vi "CalcCam4Build.vi"(11 "BuildSize":dbl) -> (3 "CamOut":T1)   [LabVIEW 2014]
uses:
  TypeDefs/Camera.ctl
  <vilib>/Utility/miscctls.llb/LV3DPointTypeDef.ctl
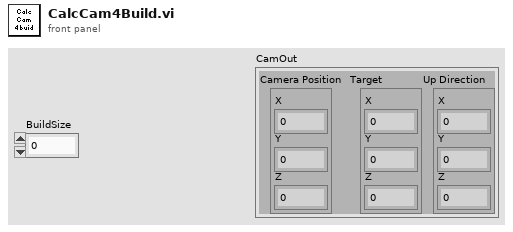
[diagram p1: front panel]
types:
  T1 = typedef "Camera.ctl" = cluster{"Camera Position":T2, "Target":T2, "Up Direction":T2}
  T2 = typedef "LV3DPointTypeDef.ctl" = cluster{"X":sgl, "Y":sgl, "Z":sgl}
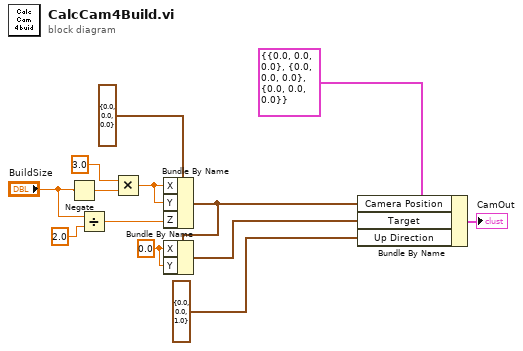
[diagram p0: block diagram]
diagram:
  w10 = sgl 0.0 ("X")
  n1 = Negate(x="BuildSize") -> (-x=w9:dbl)
  n2 = Divide(x="BuildSize", y=2.0) -> (x/y=w11:dbl)
  n3 = Multiply(x=3.0, y=w9) -> (x*y=w7:dbl)
  n4 = Bundle By Name(cluster=T2 {"X"=0.0, "Y"=0.0, "Z"=0.0} ("Camera Position"), "X"=w7, "Y"=w7, "Z"=w11) -> (w5:T2)
  n5 = Bundle By Name(cluster=w5, "X"=w10, "Y"=w10) -> (w4:T2)
  n6 = Bundle By Name(cluster=T1 {"Camera Position"={"X"=0.0, "Y"=0.0, "Z"=0.0}, "Target"={"X"=0.0, "Y"=0.0, "Z"=0.0}, "Up Direction"={"X"=0.0, "Y"=0.0, "Z"=0.0}} ("Camera"), "Camera Position"=w5, "Target"=w4, "Up Direction"=T2 {"X"=0.0, "Y"=0.0, "Z"=1.0}) -> (→"CamOut":T1)
